vi "JoystickRecorder.vi"(10 "GantryButtons":bool[](array[boolean])=[FALSE, FALSE, FALSE, FALSE, FALSE, FALSE, FALSE, FALSE, FALSE, FALSE, FALSE], 11 "JoystickValues":dbl[](array[numeric])) -> ()   [LabVIEW 2014]
uses:
  <vilib>/Analysis/Matrix/Datatypes/RealMatrix.ctl
  <vilib>/Analysis/Matrix/NI_Matrix.lvlib
panel:
  out "GantryButtonsOut":T1
  out "JoystickRecorded":T1
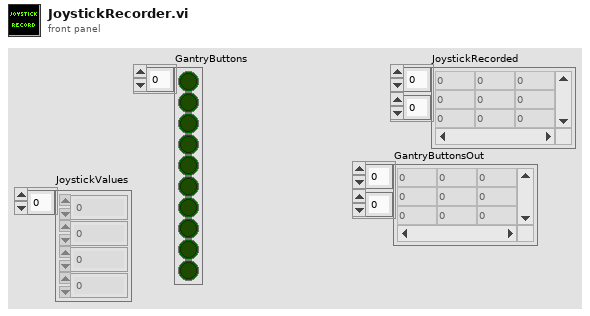
[diagram p1: front panel]
types:
  T1 = typedef "NI_Matrix.lvlib/RealMatrix.ctl" = dbl[][]
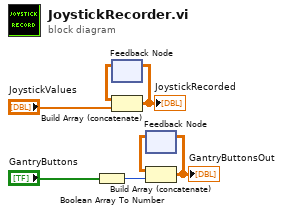
[diagram p0: block diagram]
diagram:
  n1 = Boolean Array To Number(Boolean array="GantryButtons") -> (number=w2:u32)
  n2 = feedback #1() -> (w5:T1)  [unwired: 1 in]
  n3 = Build Array (concatenate)(w5, "JoystickValues") -> (w6:T1)
  "JoystickRecorded" <- w6
  n4 = feedback-in #1(w6) -> ()
  n5 = feedback #2() -> (w3:T1)  [unwired: 1 in]
  n6 = Build Array (concatenate)(w3, w2) -> (w1:T1)
  "GantryButtonsOut" <- w1
  n7 = feedback-in #2(w1) -> ()
